vi "Update Configuration.vi"(8 "error in (no error)":errorcluster, 11 "Random Path":path) -> (0 "error out":errorcluster)   [LabVIEW 2020, in "Performance Monitor UI.lvlib" / "Configuration.lvlib"]
doc: "This VI is used where a module updates its own data, and the configuration page(s) needs to reflect the latest data from the module.\n_____\nBased on DCFG Project Template 1.0.0.21.\n____\nPeloton Config 1.0.0.2\nCopyright (c) 2022, Peloton"
uses:
  Configuration.lvlib
  Configuration DVR Global.vi
  <vilib>/Peloton/Peloton Config/Libraries/DCFG Framework/Peloton_DCFG Framework.lvlib
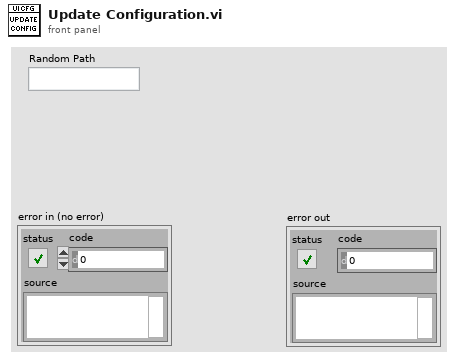
[diagram p1: front panel]
types:
  T1 = typedef "Rename As Application UI.lvlib/Configuration.lvlib/Configuration--cluster.ctl" = cluster{"Random Path":path}
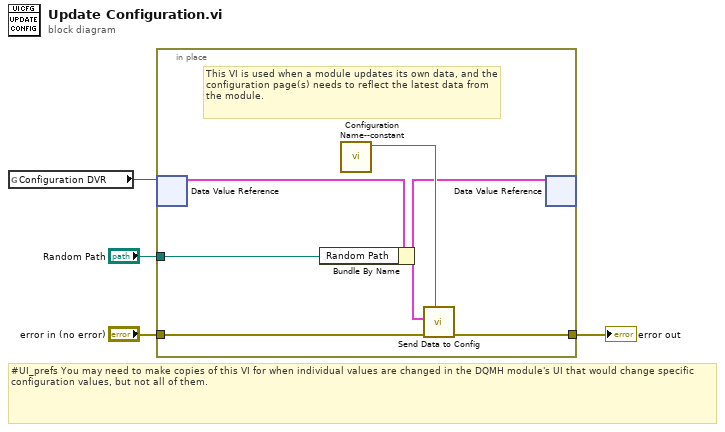
[diagram p0: block diagram]
diagram:
  # "#UI_prefs You may need to make copies of this VI for when individual values are changed in the DQMH module's UI that would change specific configuration values, but not all of them."
  n1 = global read "Configuration DVR Global.vi" "Configuration DVR"() -> (w4:refnum<data-value>)
  n2 = in-place {
    in-place-border: "Random Path" -> [w7]
    in-place-border: "error in (no error)" -> [w6]
    in-place-border: [w5] -> w1
    # "This VI is used when a module updates its own data, and the configuration page(s) needs to reflect the latest data from the module."
    n3 = in-place-dvr #1(w4) -> (w9:T1)  [unwired: 1 out]
    n4 = Bundle By Name(cluster=w9, "Random Path"=w7) -> (w8:T1)
    n5 = call "Configuration Name--constant.vi"() -> ("Configuration Name"=w10:string)  [unwired: 11 in]
    n6 = call <vilib>:"Send Data to Config.vi"("Page"=w10, "error in (no error)"=w6, "New Data"=w8) -> ("error out"=w5:errorcluster)  [unwired: 8 in]
    n7 = in-place-dvr #1(w8) -> ()  [unwired: 2 out]
  }
  "error out" <- w1
